vi "TCP Write.vi"(8 "error in (no error)":errorcluster caption="错误输入（无错误）", 10 "*(类型 *) &x":string, 11 "连接ID":refnum<k5>) -> (0 "错误输出":errorcluster, 3 "连接ID输出":refnum<k5>)   [LabVIEW 2017]
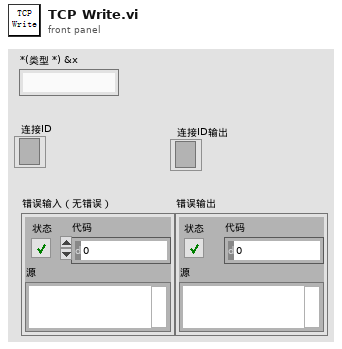
[diagram p1: front panel]
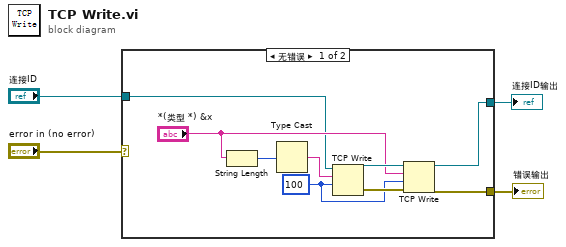
[diagram p0: block diagram]
diagram:
  n1 = case shown="无错误" "error in (no error)" {
    selector: "error in (no error)" -> [_ w15]
    tunnel: [w8 w15] -> w3
    tunnel: "连接ID" -> [w6 w14]
    tunnel: [w5 w14] -> w1
    frame No Error {
      w9 = 100 ("超时毫秒(25000)")
      n2 = String Length(string="*(类型 *) &x") -> (length=w11:i32)
      n3 = Type Cast(x=w11) -> (*(type *) &x=w12:string)  [unwired: 1 in]
      n4 = TCP Write(connection ID=w6, data in=w12, 9:w9) -> (connection ID out=w13:refnum<k5>, error out=w10:errorcluster)  [unwired: 1 in, 1 out]
      n5 = TCP Write(connection ID=w13, data in="*(类型 *) &x", error in (no error)=w10, 9:w9) -> (connection ID out=w5:refnum<k5>, error out=w8:errorcluster)  [unwired: 1 out]
    }
    frame Error {
    }
  }
  "错误输出" <- w3
  "连接ID输出" <- w1
